vi "ConvertStringTimeToTimeStamp.vi"(11 "StringTime in":string) -> (3 "TimeStamp out":timestamp format="%<%H:%M:%S%1u>T")   [LabVIEW 2018, in "Library-DataConvert.lvlib"]
uses:
  Library-DataConvert.lvlib
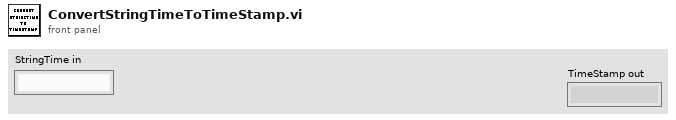
[diagram p1: front panel]
types:
  T1 = typedef "LVDateTimeRec.ctl" = cluster{"소수점 초":dbl, "초":i32, "분":i32, "시":i32, "월중의 일":i32, "월":i32, "연도":i32, "주중의 일":i32, "연중의 일":i32, "일광 절약 시간":i32}
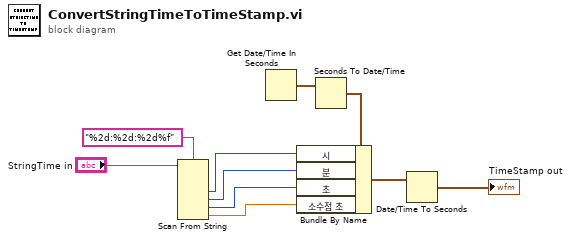
[diagram p0: block diagram]
diagram:
  n1 = Scan From String(format string="%2d:%2d:%2d%f" ("포맷 문자열"), input string="StringTime in") -> (output 1=w7:i32, output 2=w6:i32, output 3=w5:i32, output 4=w4:dbl)  [unwired: 6 in, 3 out]
  n2 = Get Date/Time In Seconds() -> (seconds since 1Jan1904=w10:timestamp)
  n3 = Seconds To Date/Time(time stamp (now)=w10) -> (date time rec=w3:T1)  [unwired: 1 in]
  n4 = Bundle By Name(cluster=w3, "시"=w7, "분"=w6, "초"=w5, "소수점 초"=w4) -> (w2:T1)
  n5 = Date/Time To Seconds(2:w2) -> (0:→"TimeStamp out":timestamp)  [unwired: 1 in]
